vi "Load Available Components.vi"(8 "error in (no error)":errorcluster, 11 "components directory":path) -> (0 "error out":errorcluster, 3 "component paths":path[](array[path]))   [LabVIEW 2017, in "DSF System Explorer.lvlib"]
uses:
  DSF System Explorer.lvlib
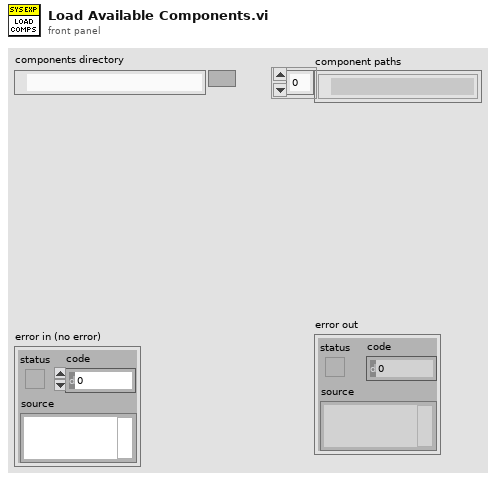
[diagram p1: front panel]
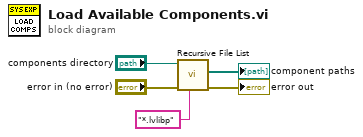
[diagram p0: block diagram]
diagram:
  n1 = call <vilib>:"Recursive File List.vi"("pattern"="*.lvlibp", "error in (no error)"="error in (no error)", "Folder Path"="components directory") -> ("error out"=→"error out":errorcluster, "All Files in Dir"=→"component paths":path[])  [unwired: 4 in, 3 out]
